vi "Control Mode Write Single.vi"(8 "error in":errorcluster, 9 "Channel Index":i32, 10 "Control Mode STS":u16, 11 "Power Supply In":refnum<class "Power Supply.lvclass">) -> (0 "error out":errorcluster, 3 "Power Supply Out":refnum<class "Power Supply.lvclass">)   [LabVIEW 2023, in "Power Supply.lvclass"]
uses:
  Power Supply.lvclass
  Low Level Capabilities/Control Mode/Control Mode.lvclass
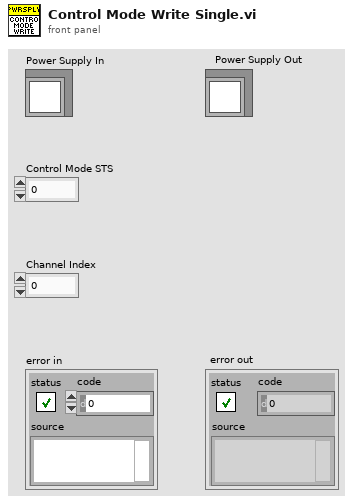
[diagram p1: front panel]
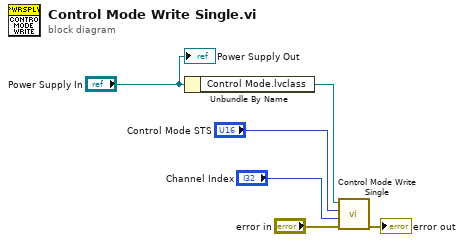
[diagram p0: block diagram]
diagram:
  n1 = Unbundle By Name("Power Supply In") -> ("Control Mode.lvclass"=w5:refnum<class "Control Mode.lvclass">)
  n2 = call-dynamic "Control Mode Write Single.vi"("error in"="error in", "Channel Index"="Channel Index", "Control Mode STS"="Control Mode STS", "Control Mode in"=w5) -> ("error out"=→"error out":errorcluster)  [unwired: 6 in, 1 out]
  "Power Supply Out" <- "Power Supply In"
